vi "Begin.vi"(8 "error in":errorcluster) -> (0 "error out":errorcluster)   [LabVIEW 2020]
doc: "Called before other user functions, this VI is expected to open initial I/O refnums, load in file data, and do all program initialization. Notice that the <B>error out</B> terminal is simply used for data flow. Wiring it to other structures or subVIs ensures that this VI runs first."
uses:
  <vilib>/Rock Robotics/WPI/DriverStation/WPI_DriverStationRobotMode2.ctl
  <vilib>/Rock Robotics/WPI/Joystick/WPI_JoystickDeviceEnum.ctl
  <vilib>/Rock Robotics/SystemInterfaces/DIO/FPGA_DIOChannel.ctl
  <vilib>/Rock Robotics/SystemInterfaces/DIO/FPGA_DIOPWMChannel.ctl
  Robot Global Data.vi
  <vilib>/Rock Robotics/Network Tables/NT Write String Array.vi
  <vilib>/Rock Robotics/WPI/Counter/WPI_CounterDigitalInputToDigitalSource.vi
  SUB VIs/TOGGLE GLOBAL.vi
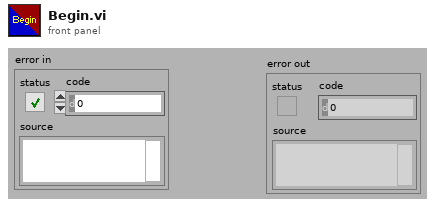
[diagram p1: front panel]
types:
  T1 = typedef "FPGA_DIOChannel.ctl" = enum8{"DIO 0", "DIO 1", "DIO 2", "DIO 3", "DIO 4", "DIO 5", "DIO 6", "DIO 7", "DIO 8", "DIO 9", "DIO MXP 0", "DIO MXP 1", "DIO MXP 2", "DIO MXP 3", "DIO MXP 4", "DIO MXP 5", "DIO MXP 6", "DIO MXP 7", "DIO MXP 8", "DIO MXP 9", "DIO MXP 10", "DIO MXP 11", "DIO MXP 12", "DIO MXP 13", "DIO MXP 14", "DIO MXP 15", "SPI Port CS1", "SPI Port CS2", "SPI Port CS3", "SPI Port MISO", "SPI Port MOSI", "Invalid"}
  T2 = typedef "WPI_JoystickDeviceEnum.ctl" = enum16{"USB 0", "USB 1", "USB 2", "USB 3", "USB 4", "USB 5"}
  T3 = typedef "FPGA_DIOPWMChannel.ctl" = enum8{"PWM 0", "PWM 1", "PWM 2", "PWM 3", "PWM 4", "PWM 5", "PWM 6", "PWM 7", "PWM 8", "PWM 9", "PWM MXP 0", "PWM MXP 1", "PWM MXP 2", "PWM MXP 3", "PWM MXP 4", "PWM MXP 5", "PWM MXP 6", "PWM MXP 7", "PWM MXP 8", "PWM MXP 9", "Invalid"}
  T4 = typedef "WPI_DriverStationRobotMode2.ctl" = enum16{"Autonomous Disabled", "Autonomous Enabled", "Teleop Disabled", "Teleop Enabled", "Disconnected", "Finish", "Test Disabled", "Test Enabled", "Emergency Stopped"}
  T5 = typedef "WPI_JoystickDevRef.ctl" = cluster{"Device":T2}
  T6 = typedef "WPI_DigitalInputDevRef.ctl" = cluster{"DevStatus":errorcluster, "DIO Channel":T1}
  T7 = typedef "FPGA_CounterEncoderSourceConvertionLVSourceType.ctl" = cluster{"DevStatus":errorcluster, "AnalogTriggerMode?":bool, "DigitalMode":cluster{"DIO Channel":T8}, "AnalogTriggerMode":cluster{"AnalogTriggerIndex":T9, "OutputType":T10}}
  T8 = typedef "FPGA_DIODigitalSourceChannel.ctl" = enum8{"DIO 0", "DIO 1", "DIO 2", "DIO 3", "DIO 4", "DIO 5", "DIO 6", "DIO 7", "DIO 8", "DIO 9", "DIO MXP 0", "DIO MXP 1", "DIO MXP 2", "DIO MXP 3", "DIO MXP 4", "DIO MXP 5", "DIO MXP 6", "DIO MXP 7", "DIO MXP 8", "DIO MXP 9", "DIO MXP 10", "DIO MXP 11", "DIO MXP 12", "DIO MXP 13", "DIO MXP 14", "DIO MXP 15", "SPI Port CS1", "SPI Port CS2", "SPI Port CS3", "SPI Port MISO", "SPI Port MOSI", "Disabled"}
  T9 = typedef "FPGA_AnalogTriggerIndex.ctl" = enum8{"Trig 0", "Trig 1", "Trig 2", "Trig 3", "Trig 4", "Trig 5", "Trig 6", "Trig 7", "Invalid"}
  T10 = typedef "FPGA_AnalogTriggerOutType.ctl" = enum16{"InWindow", "TriggerState", "Rising", "Falling"}
  T11 = typedef "WPI_EncoderDevRef.ctl" = cluster{"DevStatus":errorcluster, "EncoderIndex":T12, "CounterIndex":T13, "DistancePerCount":dbl, "Decoding Type":T14}
  T12 = typedef "FPGA_EncoderIdx.ctl" = enum8{"Enc 0", "Enc 1", "Enc 2", "Enc 3", "Enc 4", "Enc 5", "Enc 6", "Enc 7", "Invalid"}
  T13 = typedef "FPGA_CounterCtrSystemIndex.ctl" = enum8{"Ctr 0", "Ctr 1", "Ctr 2", "Ctr 3", "Ctr 4", "Ctr 5", "Ctr 6", "Ctr 7", "Invalid"}
  T14 = typedef "WPI_EncoderType.ctl" = enum16{"1x", "2x", "4x"}
  T15 = typedef "WPI_MotorControlDeviceRef.ctl" = cluster{"DeviceStatus":errorcluster, "Type":T16, "PWM":cluster{"PWM Channel":T3, "DeadBand":T17}, "CAN":cluster{"Device Number":u8, "SetOutput VI Ref":variant, "GetOutput VI Ref":variant, "Enable VI Ref":variant, "Disable VI Ref":variant, "Data":variant}, "Invert":bool, "DIO PWM":cluster{"PWM \"Enable\" Channel":T3, "DIOChannel":T1, "PWM Rate":dbl}}
  T16 = typedef "WPI_MotorControlType.ctl" = enum16{"PWM", "CAN", "DIO PWM"}
  T17 = typedef "WPI_PWMDeadband.ctl" = cluster{"Name":string, "maxPositivePwm":i32, "minPositivePwm":i32, "centerPwm":i32, "maxNegativePwm":i32, "minNegativePwm":i32, "angularRange":u16}
  T18 = typedef "CTRE_PigeonIMU_DeviceRef.ctl" = cluster{"DeviceStatus":errorcluster, "Device Number":u8, "Type":T19, "Device ID":u32, "Handle":u64, "UsageFrame":u32, "Library Path":path}
  T19 = typedef "CTRE_PigeonIMU_ConnectionType.ctl" = u32
  T20 = typedef "WPI_ServoDeviceRef.ctl" = cluster{"DeviceStatus":errorcluster, "PWM Channel":T3, "DeadBand":T17}
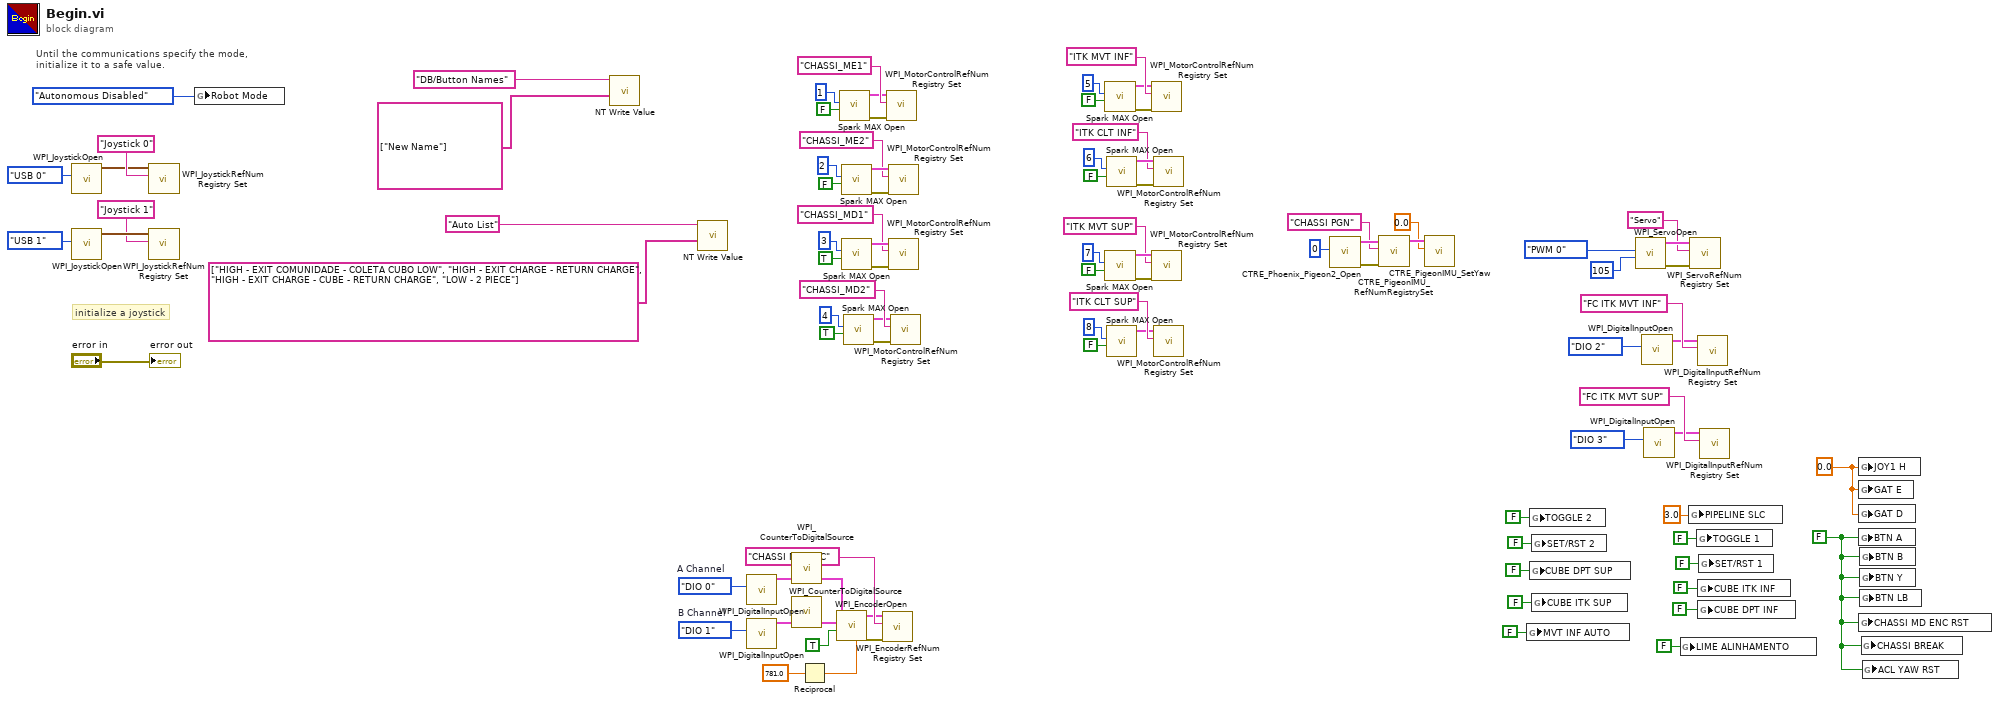
[diagram p0: block diagram]
diagram:
  w2 = FALSE ("BTN A")
  w3 = 0.0 ("JOY1 H")
  w22 = FPGA_DIOChannel."DIO 1"  # B Channel
  w23 = FPGA_DIOChannel."DIO 0"  # A Channel
  # "initialize a joystick"
  # "Until the communications specify the mode,\ninitialize it to a safe value."
  n1 = call <vilib>:"WPI_JoystickOpen.vi"("JoystickDevice"=WPI_JoystickDeviceEnum."USB 0") -> ("JoystickDevRef"=w91:T5)  [unwired: 10 in]
  n2 = call <vilib>:"WPI_JoystickOpen.vi"("JoystickDevice"=WPI_JoystickDeviceEnum."USB 1") -> ("JoystickDevRef"=w27:T5)  [unwired: 10 in]
  n3 = call <vilib>:"WPI_JoystickRefNum Registry Set.vi"("refnum name"="Joystick 0", "JoystickDevRef"=w91) -> ()  [unwired: 8 in, 2 out]
  n4 = call <vilib>:"WPI_JoystickRefNum Registry Set.vi"("refnum name"="Joystick 1", "JoystickDevRef"=w27) -> ()  [unwired: 8 in, 2 out]
  n5 = global write "Robot Global Data.vi" "Robot Mode"(WPI_DriverStationRobotMode2."Autonomous Disabled" ("Robot Mode")) -> ()
  n6 = call-poly <vilib>:"NT Write Value.vi"("value"=string[] ["New Name"], "name"="DB/Button Names" ("Name")) -> ()  [unwired: 9 in, 1 out]
  n7 = call-poly <vilib>:"NT Write Value.vi"("value"=string[] ["HIGH - EXIT COMUNIDADE - COLETA CUBO LOW", "HIGH - EXIT CHARGE - RETURN CHARGE", "HIGH - EXIT CHARGE - CUBE - RETURN CHARGE", "LOW - 2 PIECE"] ("String Array"), "name"="Auto List" ("Name")) -> ()  [unwired: 9 in, 1 out]
  n8 = call <vilib>:"WPI_DigitalInputOpen.vi"("DIO Channel"=w23) -> ("DigitalInputDevRef"=w25:T6)  [unwired: 1 in, 9 out]
  n9 = call <vilib>:"WPI_DigitalInputOpen.vi"("DIO Channel"=w22) -> ("DigitalInputDevRef"=w24:T6)  [unwired: 1 in, 9 out]
  n10 = call-poly <vilib>:"WPI_CounterToDigitalSource.vi"("DigitalInputDevRef"=w25) -> ("Digital Source"=w21:T7)  [unwired: 6 out]
  n11 = call-poly <vilib>:"WPI_CounterToDigitalSource.vi"("DigitalInputDevRef"=w24) -> ("Digital Source"=w20:T7)  [unwired: 6 out]
  n12 = Reciprocal(x=781.0) -> (1/x=w14:dbl)
  n13 = call <vilib>:"WPI_EncoderOpen.vi"("DistancePerCount"=w14, "Invert Direction (False)"=TRUE, "BSource"=w20, "ASource"=w21) -> ("error out"=w17:errorcluster, "EncoderDevRef"=w18:T11)  [unwired: 6 in]
  n14 = call <vilib>:"Spark MAX Open.vi"("Invert"=FALSE, "Device Number"=u8 1) -> ("error out"=w81:errorcluster, "MotorControlDeviceRef"=w82:T15)  [unwired: 8 in]
  n15 = call <vilib>:"Spark MAX Open.vi"("Invert"=FALSE, "Device Number"=u8 2) -> ("error out"=w80:errorcluster, "MotorControlDeviceRef"=w79:T15)  [unwired: 8 in]
  n16 = call <vilib>:"Spark MAX Open.vi"("Invert"=TRUE, "Device Number"=u8 3) -> ("error out"=w76:errorcluster, "MotorControlDeviceRef"=w75:T15)  [unwired: 8 in]
  n17 = call <vilib>:"Spark MAX Open.vi"("Invert"=TRUE, "Device Number"=u8 4) -> ("error out"=w69:errorcluster, "MotorControlDeviceRef"=w70:T15)  [unwired: 8 in]
  n18 = call <vilib>:"WPI_EncoderRefNum Registry Set.vi"("error in (no error)"=w17, "refnum name"="CHASSI MD ENC", "EncoderDevRef"=w18) -> ()  [unwired: 7 in, 2 out]
  n19 = call <vilib>:"WPI_MotorControlRefNum Registry Set.vi"("error in (no error)"=w81, "refnum name"="CHASSI_ME1", "MotorControlDevRef"=w82) -> ()  [unwired: 7 in, 2 out]
  n20 = call <vilib>:"WPI_MotorControlRefNum Registry Set.vi"("error in (no error)"=w80, "refnum name"="CHASSI_ME2", "MotorControlDevRef"=w79) -> ()  [unwired: 7 in, 2 out]
  n21 = call <vilib>:"WPI_MotorControlRefNum Registry Set.vi"("error in (no error)"=w76, "refnum name"="CHASSI_MD1", "MotorControlDevRef"=w75) -> ()  [unwired: 7 in, 2 out]
  n22 = call <vilib>:"WPI_MotorControlRefNum Registry Set.vi"("error in (no error)"=w69, "refnum name"="CHASSI_MD2", "MotorControlDevRef"=w70) -> ()  [unwired: 7 in, 2 out]
  n23 = call <vilib>:"Spark MAX Open.vi"("Invert"=FALSE, "Device Number"=u8 5) -> ("error out"=w55:errorcluster, "MotorControlDeviceRef"=w56:T15)  [unwired: 8 in]
  n24 = call <vilib>:"Spark MAX Open.vi"("Invert"=FALSE, "Device Number"=u8 7) -> ("error out"=w42:errorcluster, "MotorControlDeviceRef"=w41:T15)  [unwired: 8 in]
  n25 = call <vilib>:"Spark MAX Open.vi"("Invert"=FALSE, "Device Number"=u8 6) -> ("error out"=w62:errorcluster, "MotorControlDeviceRef"=w61:T15)  [unwired: 8 in]
  n26 = call <vilib>:"Spark MAX Open.vi"("Invert"=FALSE, "Device Number"=u8 8) -> ("MotorControlDeviceRef"=w36:T15)  [unwired: 8 in, 1 out]
  n27 = call <vilib>:"WPI_MotorControlRefNum Registry Set.vi"("error in (no error)"=w55, "refnum name"="ITK MVT INF", "MotorControlDevRef"=w56) -> ()  [unwired: 7 in, 2 out]
  n28 = call <vilib>:"WPI_MotorControlRefNum Registry Set.vi"("error in (no error)"=w42, "refnum name"="ITK MVT SUP", "MotorControlDevRef"=w41) -> ()  [unwired: 7 in, 2 out]
  n29 = call <vilib>:"WPI_MotorControlRefNum Registry Set.vi"("error in (no error)"=w62, "refnum name"="ITK CLT INF", "MotorControlDevRef"=w61) -> ()  [unwired: 7 in, 2 out]
  n30 = call <vilib>:"WPI_MotorControlRefNum Registry Set.vi"("refnum name"="ITK CLT SUP", "MotorControlDevRef"=w36) -> ()  [unwired: 8 in, 2 out]
  n31 = call <vilib>:"CTRE_Phoenix_Pigeon2_Open.vi"("Device Number"=u8 0) -> ("error out"=w51:errorcluster, "PigeonIMUDevRef"=w50:T18)  [unwired: 9 in]
  n32 = call <vilib>:"CTRE_PigeonIMU_RefNumRegistrySet.vi"("error in (no error)"=w51, "refnum name"="CHASSI PGN", "PigeonIMUDevRef"=w50) -> ("PigeonIMUDevRef"=w49:T18)  [unwired: 7 in, 1 out]
  n33 = call <vilib>:"CTRE_PigeonIMU_SetYaw.vi"("Value"=0.0, "PigeonIMUDevRef"=w49) -> ()  [unwired: 8 in, 2 out]
  n34 = global write "Robot Global Data.vi" "MVT INF AUTO"(FALSE ("MVT INF AUTO")) -> ()
  n35 = global write "TOGGLE GLOBAL.vi" "TOGGLE 2"(FALSE ("TOGGLE 2")) -> ()
  n36 = global write "Robot Global Data.vi" "CUBE DPT SUP"(FALSE ("CUBE DPT SUP")) -> ()
  n37 = global write "TOGGLE GLOBAL.vi" "SET/RST 2"(FALSE ("SET/RST 2")) -> ()
  n38 = global write "Robot Global Data.vi" "CUBE ITK SUP"(FALSE ("CUBE ITK SUP")) -> ()
  n39 = call <vilib>:"WPI_ServoOpen.vi"("Angular Range"=u16 105, "PWM Channel"=FPGA_DIOPWMChannel."PWM 0") -> ("error out"=w31:errorcluster, "ServoDeviceRef"=w30:T20)  [unwired: 8 in]
  n40 = call <vilib>:"WPI_DigitalInputOpen.vi"("DIO Channel"=FPGA_DIOChannel."DIO 2") -> ("DigitalInputDevRef"=w52:T6)  [unwired: 9 in, 1 out]
  n41 = call <vilib>:"WPI_DigitalInputOpen.vi"("DIO Channel"=FPGA_DIOChannel."DIO 3") -> ("DigitalInputDevRef"=w43:T6)  [unwired: 9 in, 1 out]
  n42 = global write "Robot Global Data.vi" "LIME ALINHAMENTO"(FALSE ("LIME ALINHAMENTO")) -> ()
  n43 = global write "Robot Global Data.vi" "PIPELINE SLC"(3.0 ("PIPELINE SLC")) -> ()
  n44 = call <vilib>:"WPI_ServoRefNum Registry Set.vi"("error in (no error)"=w31, "refnum name"="Servo", "ServoDeviceRef"=w30) -> ()  [unwired: 7 in, 2 out]
  n45 = global write "TOGGLE GLOBAL.vi" "TOGGLE 1"(FALSE ("TOGGLE 2")) -> ()
  n46 = call <vilib>:"WPI_DigitalInputRefNum Registry Set.vi"("refnum name"="FC ITK MVT INF", "DigitalInputDevRef"=w52) -> ()  [unwired: 8 in, 2 out]
  n47 = global write "Robot Global Data.vi" "CUBE ITK INF"(FALSE ("CUBE ITK SUP")) -> ()
  n48 = global write "Robot Global Data.vi" "CUBE DPT INF"(FALSE ("CUBE DPT SUP")) -> ()
  n49 = global write "TOGGLE GLOBAL.vi" "SET/RST 1"(FALSE ("SET/RST 2")) -> ()
  n50 = call <vilib>:"WPI_DigitalInputRefNum Registry Set.vi"("refnum name"="FC ITK MVT SUP", "DigitalInputDevRef"=w43) -> ()  [unwired: 8 in, 2 out]
  n51 = global write "Robot Global Data.vi" "JOY1 H"(w3) -> ()
  n52 = global write "Robot Global Data.vi" "GAT E"(w3) -> ()
  n53 = global write "Robot Global Data.vi" "GAT D"(w3) -> ()
  n54 = global write "Robot Global Data.vi" "BTN A"(w2) -> ()
  n55 = global write "Robot Global Data.vi" "CHASSI MD ENC RST"(w2) -> ()
  n56 = global write "Robot Global Data.vi" "BTN B"(w2) -> ()
  n57 = global write "Robot Global Data.vi" "BTN Y"(w2) -> ()
  n58 = global write "Robot Global Data.vi" "BTN LB"(w2) -> ()
  n59 = global write "Robot Global Data.vi" "CHASSI BREAK"(w2) -> ()
  n60 = global write "Robot Global Data.vi" "ACL YAW RST"(w2) -> ()
  "error out" <- "error in"
